vi "Save Macro Config.vi"(8 "error in (no error)":errorcluster, 10 "Macro Config":T1, 11 "refnum":T2) -> (0 "error out":errorcluster, 3 "refnum out":T2)   [LabVIEW 2020, in "MacroAssert.lvlib"]
doc: "Loads the macro defined by <B>Macro Name</B> from the config file defined by <B>refnum</B>."
uses:
  MacroAssert.lvlib
  <vilib>/Utility/config.llb/Config Data RefNum.ctl
  CTLs/Macro Config V3.ctl
  <vilib>/Utility/config.llb/Write Key (I32).vi
  <vilib>/Utility/config.llb/Write Key (String).vi
  <vilib>/Utility/config.llb/NI_LVConfig.lvlib
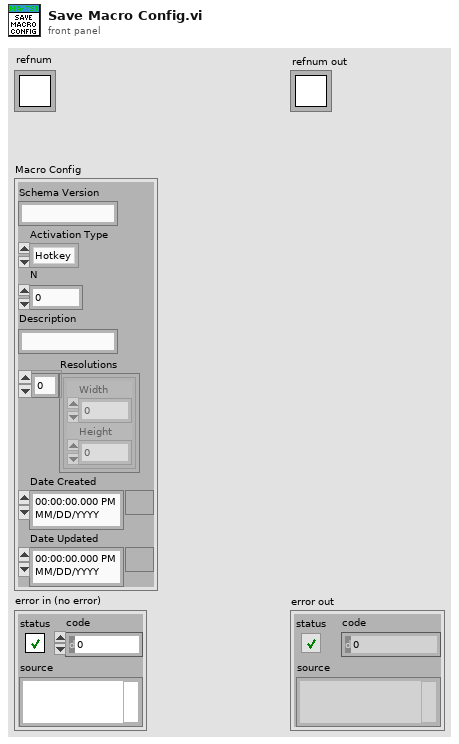
[diagram p1: front panel]
types:
  T1 = typedef "MacroAssert.lvlib/Macro Config V3.ctl" = cluster{"Schema Version":string, "Activation Type":enum32{"Hotkey", "Automatic"}, "N":i32, "Description":string, "Resolutions":cluster{"Width":i16, "Height":i16}[], "Date Created":timestamp, "Date Updated":timestamp}
  T2 = typedef "NI_LVConfig.lvlib/Config Data RefNum.ctl" = refnum<k1>
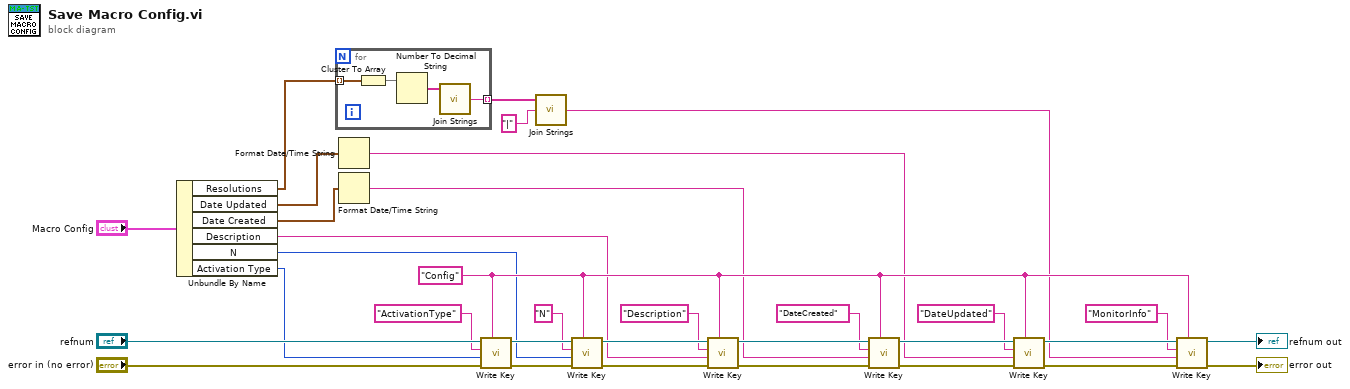
[diagram p0: block diagram]
diagram:
  w33 = "Config" ("section")
  n1 = Unbundle By Name("Macro Config") -> ("Resolutions"=w5:cluster{"Width":i16, "Height":i16}[], "Date Updated"=w6:timestamp, "Date Created"=w7:timestamp, "Description"=w10:string, "N"=w11:i32, "Activation Type"=w12:enum32{"Hotkey", "Automatic"})
  n2 = for {
    tunnel: w5 -> [w37] mode=indexing
    tunnel: [w34] -> w9 mode=indexing
    n3 = Cluster To Array(cluster=w37) -> (array=w36:i16[])
    n4 = Number To Decimal String(number=w36) -> (decimal integer string=w35:string[])  [unwired: 1 in]
    n5 = call <vilib>:"Join Strings.vi"("Strings In"=w35) -> ("String"=w34:string)  [unwired: 2 in]
  }
  n6 = Format Date/Time String(seconds (now)=w6) -> (date/time string=w3:string)  [unwired: 2 in]
  n7 = Format Date/Time String(seconds (now)=w7) -> (date/time string=w4:string)  [unwired: 2 in]
  n8 = call-poly <vilib>:"Write Key.vi"("section"=w33, "error in (no error)"="error in (no error)", "value"=w12, "key"="ActivationType", "refnum"="refnum") -> ("error out"=w22:errorcluster, "refnum out"=w29:T2)  [unwired: 4 in, 1 out]
  n9 = call <vilib>:"Join Strings.vi"("Separator (,)"="|", "Strings In"=w9) -> ("String"=w2:string)  [unwired: 1 in]
  n10 = call-poly <vilib>:"Write Key.vi"("section"=w33, "error in (no error)"=w22, "value"=w11, "key"="N", "refnum"=w29) -> ("error out"=w20:errorcluster, "refnum out"=w28:T2)  [unwired: 4 in, 1 out]
  n11 = call-poly <vilib>:"Write Key.vi"("section"=w33, "error in (no error)"=w20, "value"=w10, "key"="Description", "refnum"=w28) -> ("error out"=w18:errorcluster, "refnum out"=w27:T2)  [unwired: 4 in, 1 out]
  n12 = call-poly <vilib>:"Write Key.vi"("section"=w33, "error in (no error)"=w18, "value"=w4, "key"="DateCreated", "refnum"=w27) -> ("error out"=w16:errorcluster, "refnum out"=w26:T2)  [unwired: 4 in, 1 out]
  n13 = call-poly <vilib>:"Write Key.vi"("section"=w33, "error in (no error)"=w16, "value"=w3, "key"="DateUpdated", "refnum"=w26) -> ("error out"=w14:errorcluster, "refnum out"=w25:T2)  [unwired: 4 in, 1 out]
  n14 = call-poly <vilib>:"Write Key.vi"("section"=w33, "error in (no error)"=w14, "value"=w2, "key"="MonitorInfo", "refnum"=w25) -> ("error out"=→"error out":errorcluster, "refnum out"=→"refnum out":T2)  [unwired: 4 in, 1 out]
